vi "Verify String Input.vi"(8 "error in (no error)":errorcluster, 10 "Error Message":string, 11 "Input":string) -> (0 "error out":errorcluster, 3 "Output":string)   [LabVIEW 2024, in "Sift Client.lvlib" / "Sift Client.lvclass"]
uses:
  Sift Client.lvclass
  Sift Client.lvclass/Sift Client.ctl
  <vilib>/ErrorRing/Error Ring.xnode
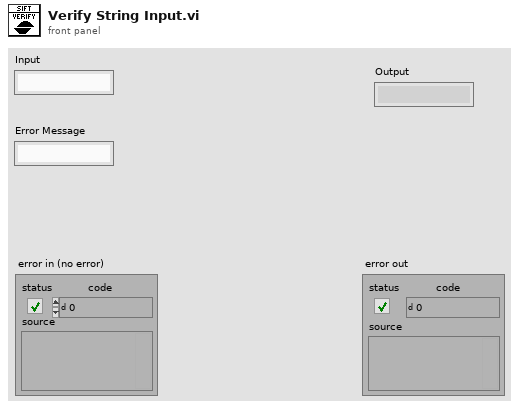
[diagram p1: front panel]
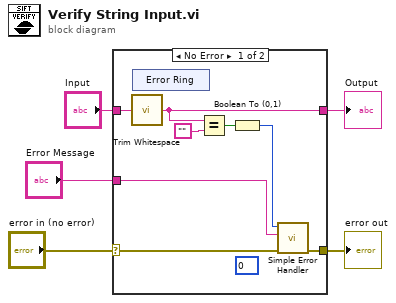
[diagram p0: block diagram]
diagram:
  n1 = case shown="No Error" "error in (no error)" {
    selector: "error in (no error)" -> [w7 w16]
    tunnel: [w8 w16] -> w4
    tunnel: "Error Message" -> [w11 _]
    tunnel: "Input" -> [w10 w15]
    tunnel: [w6 w15] -> w1
    frame No Error {
      (unwired) u16 0 items=[""]
      n2 = call <vilib>:"Trim Whitespace.vi"("string"=w10) -> ("trimmed string"=w6:string)  [unwired: 1 in]
      n3 = xnode "Error Ring"() -> ()  [unwired: 1 out]
      n4 = Equal?(x=w6, y="") -> (x = y?=w13:bool)
      n5 = Boolean To (0,1)(Boolean=w13) -> (0, 1=w12:i16)
      n6 = call <vilib>:"Simple Error Handler.vi"("error code (no error:0)"=w12, "error source (\" \")"=w11, "error in (no error)"=w7) -> ("error out"=w8:errorcluster)  [unwired: 2 in, 4 out]
    }
    frame Error {
    }
  }
  "error out" <- w4
  "Output" <- w1
